vi "Configure Data Communication Format.vi"(4 "Swap Bytes (No)":bool, 8 "error in (no error)":errorcluster, 9 "Data Selection (0: All)":u16(ring) items=["All", "Volt and Amp", "Volt", "Amp", "Volt Amp Time"], 10 "Data Type  (0: ASCII)":u16(ring) items=["ASCII", "Binary (Single Precision Real)"], 11 "VISA resource name":refnum<visa-resource-name>) -> (0 "error out":errorcluster, 3 "VISA resource name out":refnum<visa-resource-name>)   [LabVIEW 2017, in "Keithley 24XX.lvlib"]
doc: "Configures the instrument data communication format (ASCII or binary) only when the communication interface allows this. Serial only supports ASCII. Limits the data being sent over the communication line."
uses:
  Keithley 24XX.lvlib
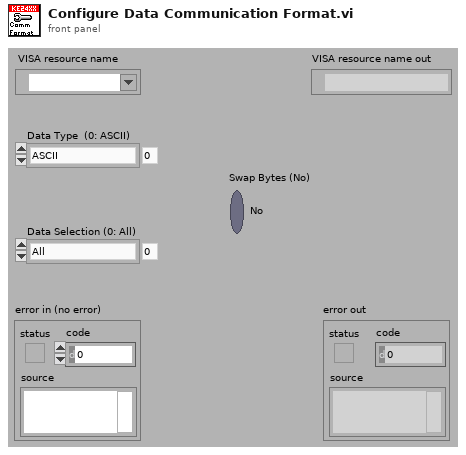
[diagram p1: front panel]
types:
  T1 = cluster{"Voltage  ":bool, "Current  ":bool, "Resistance":bool, "Time":bool, " Status ":bool}
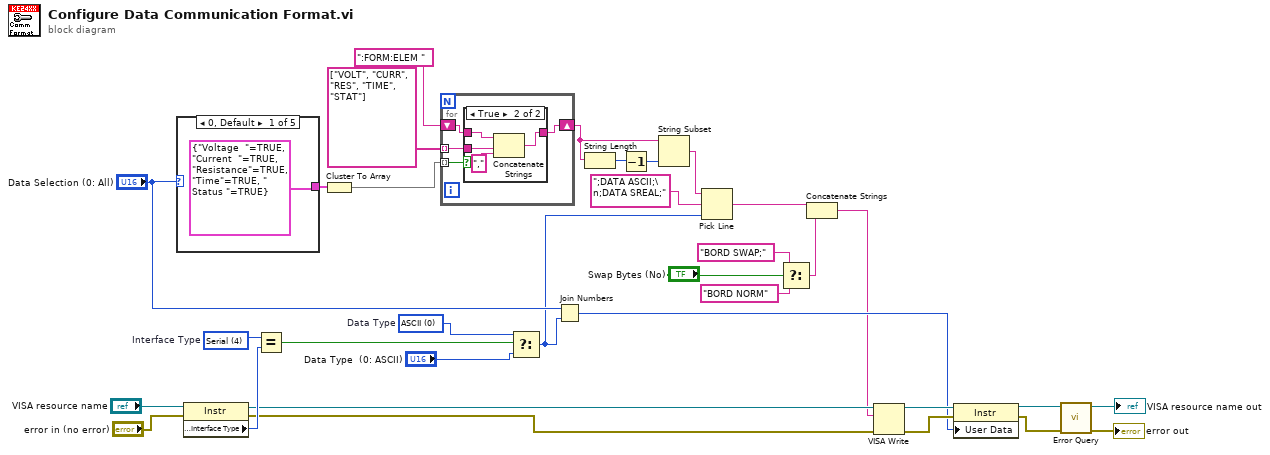
[diagram p0: block diagram]
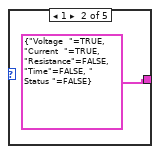
[diagram p3: hidden frame]
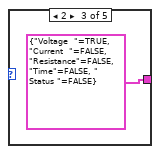
[diagram p4: hidden frame]
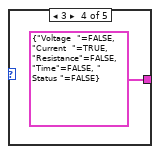
[diagram p5: hidden frame]
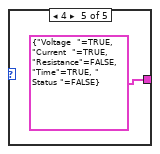
[diagram p6: hidden frame]
diagram:
  w30 = u16 0 items=["ASCII", "Binary (Single Precision Real)"]  # Data Type
  w29 = u16 4 items=["GPIB"=1, "VXI"=2, "GPIB-VXI"=3, "Serial"=4, "PXI"=5, "TCPIP"=6, "USB"=7]  # Interface Type
  n1 = case shown="0, Default" "Data Selection (0: All)" {
    tunnel: [T1 {"Voltage  "=TRUE, "Current  "=TRUE, "Resistance"=TRUE, "Time"=TRUE, " Status "=TRUE} T1 {"Voltage  "=TRUE, "Current  "=TRUE, "Resistance"=FALSE, "Time"=FALSE, " Status "=FALSE} T1 {"Voltage  "=TRUE, "Current  "=FALSE, "Resistance"=FALSE, "Time"=FALSE, " Status "=FALSE} T1 {"Voltage  "=FALSE, "Current  "=TRUE, "Resistance"=FALSE, "Time"=FALSE, " Status "=FALSE} T1 {"Voltage  "=TRUE, "Current  "=TRUE, "Resistance"=FALSE, "Time"=TRUE, " Status "=FALSE}] -> w16
    frame 0, Default {
    }
    frame 1 {
    }
    frame 2 {
    }
    frame 3 {
    }
    frame 4 {
    }
  }
  n2 = property class="Instr"(reference="VISA resource name", error in="error in (no error)") -> (reference out=w19:refnum<visa-resource-name>, error out=w18:errorcluster, "Interface Information:Interface Type"=w28:u16)
  n3 = Equal?(x=w29, y=w28) -> (x = y?=w31:bool)
  n4 = Cluster To Array(cluster=w16) -> (array=w13:bool[])
  n5 = for {
    tunnel: string[] ["VOLT", "CURR", "RES", "TIME", "STAT"] -> [w40] mode=indexing
    shift-right: [w39] -> w10
    shift-left: ":FORM:ELEM " -> [w41]
    tunnel: w13 -> [w42] mode=indexing
    n6 = case shown="True" w42 {
      tunnel: w41 -> [w43 w46]
      tunnel: w40 -> [_ w47]
      tunnel: [w43 w44] -> w39
      frame False {
      }
      frame True {
        n7 = Concatenate Strings(w46, w47, ",") -> (w44:string)
      }
    }
  }
  n8 = Select(t=w30, s=w31, f="Data Type  (0: ASCII)") -> (s? t:f=w1:u16)
  n9 = Join Numbers(hi="Data Selection (0: All)", lo=w1) -> ((hi.lo)=w24:u32)
  n10 = String Length(string=w10) -> (length=w12:i32)
  n11 = Decrement(x=w12) -> (x-1=w11:i32)
  n12 = String Subset(string=w10, length (rest)=w11) -> (substring=w9:string)  [unwired: 1 in]
  n13 = Pick Line(string ("")=w9, multi-line string=";DATA ASCII;\n;DATA SREAL;", line index=w1) -> (output string=w8:string)
  n14 = Select(t="BORD SWAP;", s="Swap Bytes (No)", f="BORD NORM") -> (s? t:f=w4:string)
  n15 = Concatenate Strings(w8, w4) -> (w3:string)
  n16 = VISA Write(VISA resource name=w19, write buffer=w3, error in (no error)=w18) -> (VISA resource name out=w26:refnum<visa-resource-name>, error out=w25:errorcluster)  [unwired: 1 out]
  n17 = property class="Instr"(reference=w26, error in=w25, "User Data"=w24) -> (reference out=w23:refnum<visa-resource-name>, error out=w22:errorcluster)
  n18 = call "Error Query.vi"("error in (no error)"=w22, "VISA resource name"=w23) -> ("error out"=→"error out":errorcluster, "VISA resource name out"=→"VISA resource name out":refnum<visa-resource-name>)  [unwired: 6 in, 2 out]
